vi "AIT 1553 - Build BM Message Properties.vi"(8 "error in (no error)":errorcluster, 10 "BM_Message":T1) -> (0 "error out":errorcluster, 1 "Tx-Rx  (T=Tx)":bool, 2 "name":string, 4 "Prop Names":string[](array[string]), 6 "Prop Values":variant[](array[variant]))   [LabVIEW 2013, in "AIT 1553 Custom Device.lvlib"]
uses:
  AIT 1553 Custom Device.lvlib
  Controls/1553_BM_Message.ctl
  Controls/1553 Param.ctl
  Controls and Global/Global.vi
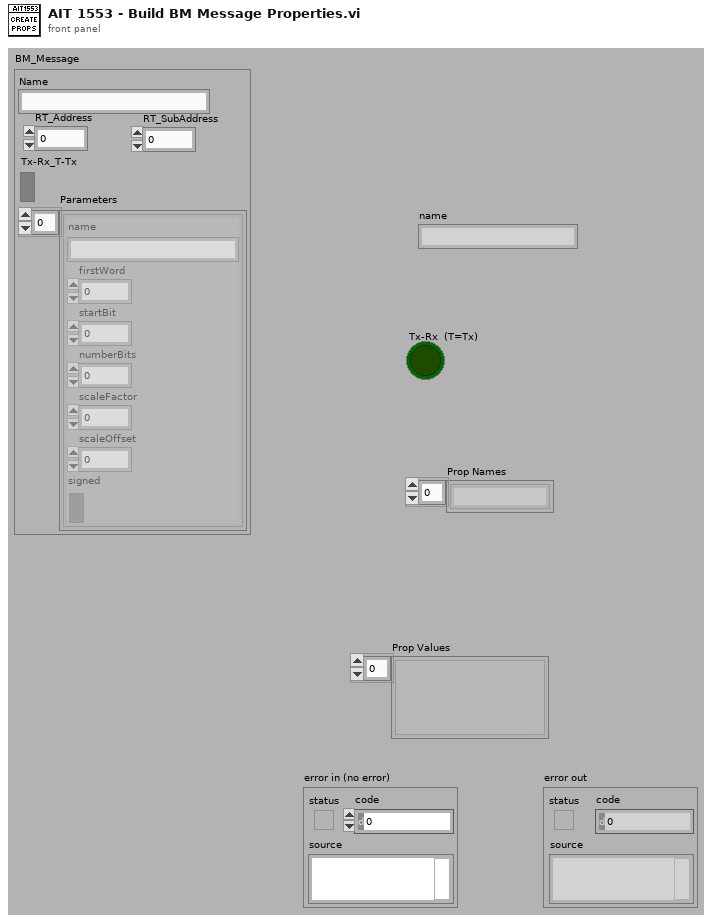
[diagram p1: front panel]
types:
  T1 = typedef "AIT 1553 Custom Device.lvlib/1553_BM_Message.ctl" = cluster{"RT_Address":u8, "RT_SubAddress":u8, "Tx-Rx_T-Tx":bool, "Parameters":T2[], "Name":string}
  T2 = typedef "AIT 1553 Custom Device.lvlib/1553 Param.ctl" = cluster{"name":string, "firstWord":i32, "startBit":i32, "numberBits":i32, "scaleFactor":dbl, "scaleOffset":dbl, "signed":bool}
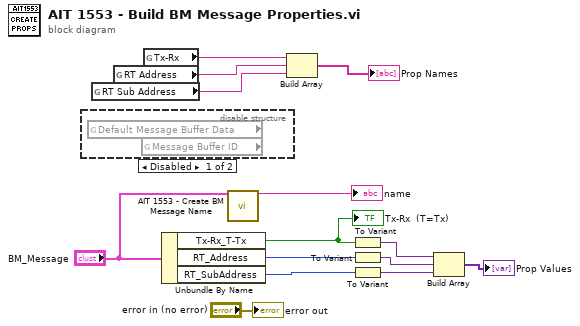
[diagram p0: block diagram]
diagram:
  n1 = disable-structure shown="Disabled" {
    frame Disabled {
      n2 = global read "Global.vi" "Default Message Buffer Data"() -> ()  [unwired: 1 out]
      n3 = global read "Global.vi" "Message Buffer ID"() -> ()  [unwired: 1 out]
    }
    frame Enabled {
    }
  }
  n4 = global read "Global.vi" "RT Sub Address"() -> (w12:string)
  n5 = global read "Global.vi" "RT Address"() -> (w3:string)
  n6 = global read "Global.vi" "Tx-Rx"() -> (w14:string)
  n7 = Unbundle By Name("BM_Message") -> ("Tx-Rx_T-Tx"=w6:bool, "RT_Address"=w7:u8, "RT_SubAddress"=w8:u8)
  "Tx-Rx  (T=Tx)" <- w6
  n8 = call "AIT 1553 - Create BM Message Name.vi"("BM_Message"="BM_Message") -> ("Message Name"=→"name":string)  [unwired: 13 in, 1 out]
  n9 = Build Array(w14, w3, w12) -> (→"Prop Names":string[])
  n10 = To Variant(anything=w6) -> (Variant=w9:variant)
  n11 = To Variant(anything=w7) -> (Variant=w10:variant)
  n12 = To Variant(anything=w8) -> (Variant=w11:variant)
  n13 = Build Array(w9, w10, w11) -> (→"Prop Values":variant[])
  "error out" <- "error in (no error)"
